vi "arm driver control.vi"(1 "Joystick Y":dbl) -> (0 "Setpoint":dbl)   [LabVIEW 2013]
panel:
  # "Control the arm with PID setpoints instead of direct motor control"
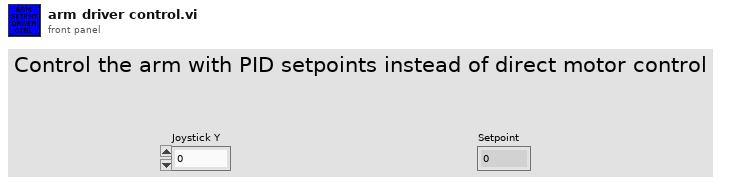
[diagram p1: front panel]
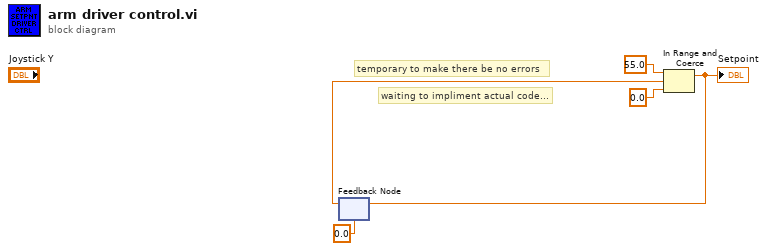
[diagram p0: block diagram]
diagram:
  # "waiting to impliment actual code..."
  # "temporary to make there be no errors"
  n1 = feedback #1(0.0 ("upper limit")) -> (w1:dbl)
  n2 = In Range and Coerce(upper limit=55.0, x=w1, lower limit=0.0) -> (coerced(x)=w3:dbl)  [unwired: 1 out]
  "Setpoint" <- w3
  n3 = feedback-in #1(w3) -> ()
